vi "液位控制.vi"() -> ()   [LabVIEW 2010]
uses:
  液位全局变量.vi
panel:
  in  "停止":bool
  in  "控制步长":dbl(knob)=0.08505482833105478 scale=0.0..1.0 scale format="%.1f"
  in  "液位设定值":dbl(slide)=81.0 scale=0.0..10.0 scale format="%.2f"
  out "容器液位":dbl(slide) scale=0.0..10.0
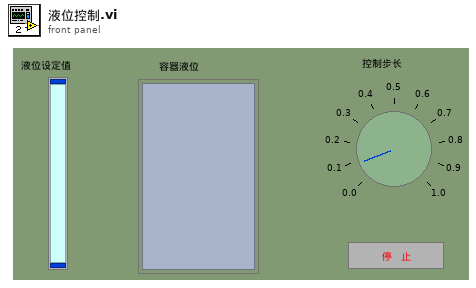
[diagram p1: front panel]
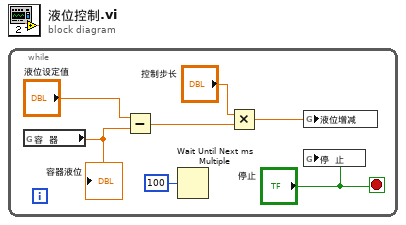
[diagram p0: block diagram]
diagram:
  n1 = while {
    stop <- "停止" stop-if-true
    n2 = global read "液位全局变量.vi" "容  器"() -> (w5:dbl)
    "容器液位" <- w5
    n3 = Subtract(x="液位设定值", y=w5) -> (x-y=w3:dbl)
    n4 = Wait Until Next ms Multiple(millisecond multiple=u32 100) -> ()  [unwired: 1 out]
    n5 = Multiply(x="控制步长", y=w3) -> (x*y=w2:dbl)
    n6 = global write "液位全局变量.vi" "液位增减"(w2) -> ()
    n7 = global write "液位全局变量.vi" "停  止"("停止") -> ()
  }
